vi "Ejemplo de aplicacion nxp.vi"() -> ()   [LabVIEW 2019, in "NXP.lvclass"]
uses:
  NXP.lvclass
  C:/Users/Luis/Documents/Ingenieria/Git_versiones/PROYECTO-FINAL-INSTRUMENTACI-N-VIRTUAL/Clase Padre/Serial Device.lvclass
  Clase Padre/Serial Device.lvclass/Serial Device.ctl
  Clase Padre/Serial Device.lvclass
panel:
  out "Response_ADC_probe":string
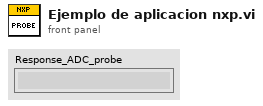
[diagram p1: front panel]
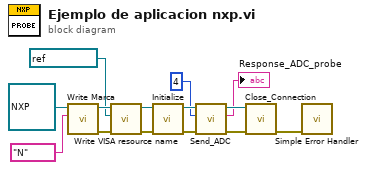
[diagram p0: block diagram]
diagram:
  n1 = call "Write Marca.vi"("Marca"="N", "Serial Device in"=refnum<class "NXP.lvclass"> refnum ("NXP.lvclass")) -> ("error out"=w13:errorcluster, "Serial Device out"=w14:refnum<class "NXP.lvclass">)  [unwired: 8 in]
  n2 = call "Write VISA resource name.vi"("error in (no error)"=w13, "VISA resource name"=refnum<visa-resource-name> "COM10", "Serial Device in"=w14) -> ("error out"=w11:errorcluster, "Serial Device out"=w12:refnum<class "NXP.lvclass">)  [unwired: 7 in]
  n3 = call-dynamic "Initialize.vi"("error in (no error)"=w11, "NXP in"=w12) -> ("error out"=w9:errorcluster, "NXP out"=w10:refnum<class "NXP.lvclass">)  [unwired: 8 in]
  n4 = call-dynamic "Send_ADC.vi"("error in (no error)"=w9, "Channel"=u8 4, "Serial Device in"=w10) -> ("error out"=w7:errorcluster, "Response"=→"Response_ADC_probe":string, "Serial Device out"=w8:refnum<class "NXP.lvclass">)  [unwired: 6 in]
  n5 = call-dynamic "Close_Connection.vi"("error in (no error)"=w7, "NXP in"=w8) -> ("error out"=w1:errorcluster)  [unwired: 8 in, 1 out]
  n6 = call <vilib>:"Simple Error Handler.vi"("error in (no error)"=w1) -> ()  [unwired: 4 in, 5 out]
